vi "fmt_formatSingleCell (String).vi"(5 "format string":string="%.6f", 7 "column":string, 8 "error in":errorcluster, 9 "data":string, 10 "row":i32, 11 "format buffer":u8[](array[numeric])=[60, 114, 111, 119, 32, 114, 61, 34, 49, 48, 52, 56, 53, 55, 54, 48, 48, 48, 48, 34, 62, 60, 99, 32, 114, 61, 34, 90, 90, 90, 90, 90, 49, 48, 52, 56, 53, 55, 54, 48, 48, 48, 48, 48, 48, 48, 34, 62, 60, 118, 62, 48, 48, 48, 48, 48, 48, 48, 48, 48, 48, 46, 48, 48, 48, 48, 48, 48, 48, 48, 48, 48, 48, 48, 48, 48, 48, 48, 48, 48, 48, 48, 48, 60, 47, 118, 62, 60, 47, 99, 62, 60, 47, 114, 111, 119, 62]) -> (0 "error out":errorcluster, 1 "formatted value length":i32, 2 "buffer size":i32, 3 "formatted buffer":u8[](array[numeric]))   [LabVIEW 2017, in "NI_ExcelFile.lvlib"]
uses:
  <vilib>/express/express shared/NI_ExcelFile/NI_ExcelFile.lvlib
  <vilib>/express/express shared/NI_ExcelFile/SubVIs/fmt_getUTF-8Text.vi
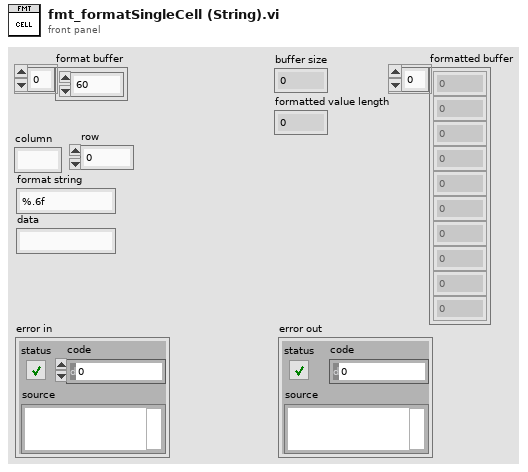
[diagram p1: front panel]
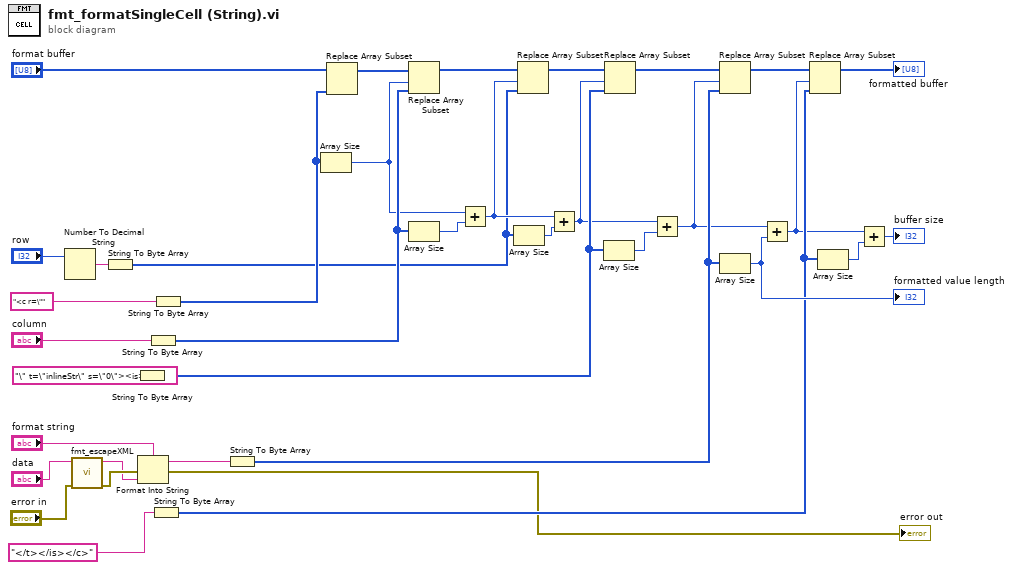
[diagram p0: block diagram]
diagram:
  n1 = Number To Decimal String(number="row") -> (decimal integer string=w11:string)  [unwired: 1 in]
  n2 = call <vilib>:"fmt_escapeXML.vi"("error in"="error in", "plain text"="data") -> ("error out"=w3:errorcluster, "xml text"=w2:string)  [unwired: 8 in]
  n3 = String To Byte Array(string=w11) -> (unsigned byte array=w10:u8[])
  n4 = String To Byte Array(string="\" t=\"inlineStr\" s=\"0\"><is><t>") -> (unsigned byte array=w26:u8[])
  n5 = Format Into String(format string="format string", error in=w3, w2) -> (resulting string=w6:string, error out=→"error out":errorcluster)  [unwired: 1 in]
  n6 = String To Byte Array(string="column") -> (unsigned byte array=w34:u8[])
  n7 = String To Byte Array(string="</t></is></c>") -> (unsigned byte array=w18:u8[])
  n8 = String To Byte Array(string="<c r=\"") -> (unsigned byte array=w31:u8[])
  n9 = String To Byte Array(string=w6) -> (unsigned byte array=w25:u8[])
  n10 = Array Size(array=w31) -> (size(s)=w14:i32)
  n11 = Replace Array Subset(array="format buffer", new element=w31) -> (w30:u8[])  [unwired: 1 in]
  n12 = Replace Array Subset(array=w30, new element=w34, index=w14) -> (w33:u8[])
  n13 = Array Size(array=w34) -> (size(s)=w24:i32)
  n14 = Add(x=w14, y=w24) -> (x+y=w28:i32)
  n15 = Array Size(array=w10) -> (size(s)=w13:i32)
  n16 = Replace Array Subset(array=w33, new element=w10, index=w28) -> (w29:u8[])
  n17 = Add(x=w28, y=w13) -> (x+y=w23:i32)
  n18 = Array Size(array=w26) -> (size(s)=w22:i32)
  n19 = Replace Array Subset(array=w29, new element=w26, index=w23) -> (w27:u8[])
  n20 = Add(x=w23, y=w22) -> (x+y=w21:i32)
  n21 = Replace Array Subset(array=w27, new element=w25, index=w21) -> (w19:u8[])
  n22 = Array Size(array=w25) -> (size(s)=w20:i32)
  "formatted value length" <- w20
  n23 = Add(x=w21, y=w20) -> (x+y=w16:i32)
  n24 = Replace Array Subset(array=w19, new element=w18, index=w16) -> (→"formatted buffer":u8[])
  n25 = Array Size(array=w18) -> (size(s)=w17:i32)
  n26 = Add(x=w16, y=w17) -> (x+y=→"buffer size":i32)
